vi "test new test.vi"(8 "error in (no error)":errorcluster, 11 "TestCase in":refnum<class "TestClass.lvclass">) -> (0 "error out":errorcluster, 3 "TestCase out":refnum<class "TestClass.lvclass">)   [LabVIEW 2013, in "TestClass.lvclass"]
uses:
  TestClass.lvclass
  Classes/TestCase/TestCase.lvclass
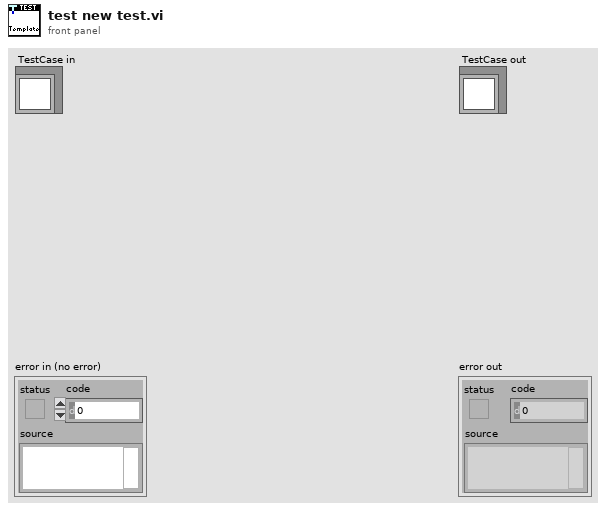
[diagram p1: front panel]
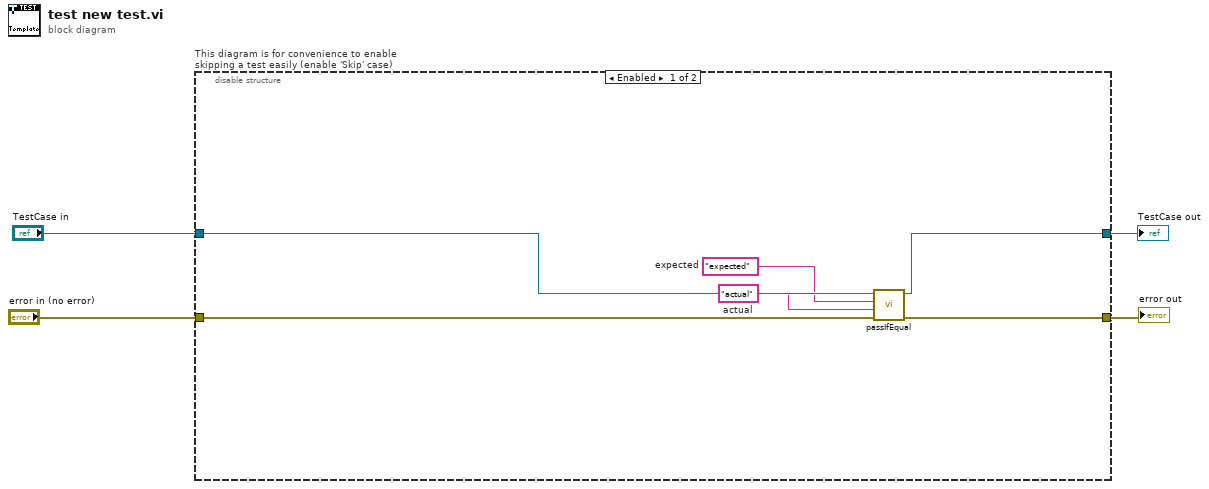
[diagram p0: block diagram]
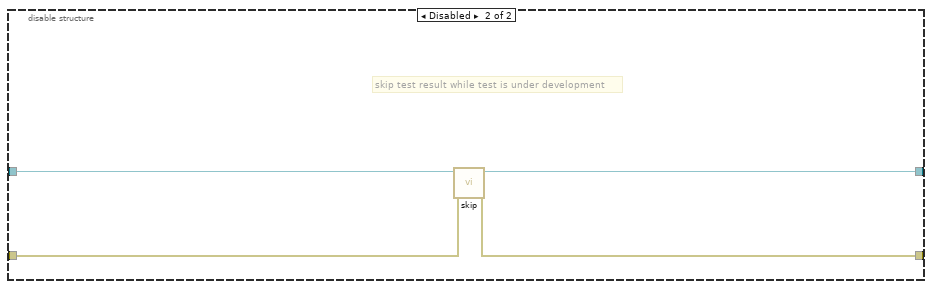
[diagram p2: hidden frame]
diagram:
  n1 = disable-structure "This diagram is for convenience to enable skipping a test easily (enable 'Skip' case)" shown="Enabled" {
    disable-tunnel: "TestCase in" -> [w10 w14]
    disable-tunnel: [w9 w12] -> w1
    disable-tunnel: [w8 w13] -> w3
    disable-tunnel: "error in (no error)" -> [w7 w11]
    frame Enabled {
      w5 = "actual"  # actual
      w6 = "expected"  # expected
      n2 = call-dynamic "passIfEqual.vi"("error in (no error)"=w7, "y"=w5, "x"=w6, "TestCase in"=w10) -> ("error out"=w8:errorcluster, "TestCase out"=w9:refnum<class "TestCase.lvclass">)  [unwired: 6 in]
    }
    frame Disabled {
      # "skip test result while test is under development"
      n3 = call "skip.vi"("error in (no error)"=w11, "TestCase in"=w14) -> ("error out"=w13:errorcluster, "TestCase out"=w12:refnum<class "TestCase.lvclass">)  [unwired: 8 in]
    }
  }
  "error out" <- w3
  "TestCase out" <- w1
